vi "Get Error Source.vi"(2 "delimiter (\"->\")":string="->", 3 "pop number":i32=2) -> (0 "dup delimiter":string, 1 "error source":string)   [LabVIEW 2019, in "CCD_camera.lvclass"]
doc: "Returns an <B>error source</B> string intended for a LabVIEW error cluster. The string contains the chain of SubVI calls from the top VI to the SubVI that caused the error.\n\nThe string building process can optionally be altered using the <B>pop number</B> parameter, which specifies how many of the most recently called subroutines should be skipped. This parameter is used to remove the internal error handling SubVIs from the resulting error source string. The default value is <B>2</B>.\n<B>Don't mess with this value, unless you know what you're doing!!</B>\n\nThe string that delimits the callers' names is by default \"<B>-></B>\", but can be modified with the <B>delimiter</B> parameter."
uses:
  CCD_camera.lvclass
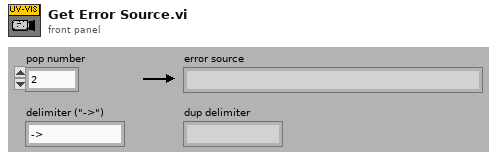
[diagram p1: front panel]
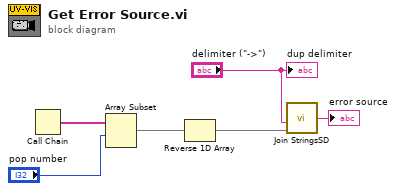
[diagram p0: block diagram]
diagram:
  n1 = Call Chain() -> (call chain=w4:string[])
  n2 = Array Subset "Array Subset"(array=w4, index="pop number") -> (w3:string[])  [unwired: 1 in]
  n3 = Reverse 1D Array(array=w3) -> (reversed array=w2:string[])
  n4 = call "Join StringsSD.vi"("string array"=w2, "delimiter (\"\")"="delimiter (\"->\")") -> ("joined string"=→"error source":string)  [unwired: 2 in]
  "dup delimiter" <- "delimiter (\"->\")"
